vi "Zone-to-color_correspondence_lookup_test_2.vi"() -> ()   [LabVIEW 2018]
uses:
  <userlib>/_OpenG.lib/array/array.llb/Sort 1D Array (U32)__ogtk.vi
  <userlib>/_OpenG.lib/array/array.llb/Index 1D Array Elements (U32)__ogtk.vi
  <vilib>/Analysis/polynomials.llb/Unique Numbers and Multiplicity (DBL).vi
  <userlib>/_OpenG.lib/array/array.llb/Index 1D Array Elements (DBL)__ogtk.vi
  <vilib>/Analysis/NI_AALPro.lvlib
panel:
  out "Seconds per MPix":dbl
  out "Amount of colors":cluster{"Amount":u32, "Color":u32}[](array[cluster])
  out "Array size":i32
  out "Image Display":T1(plugin-control)
  in  "Labyrinth path":path=path "D:/Users_Data/Dmitriy_T/Documents/Tracker/TestVI's/Labyrinth_check.png"
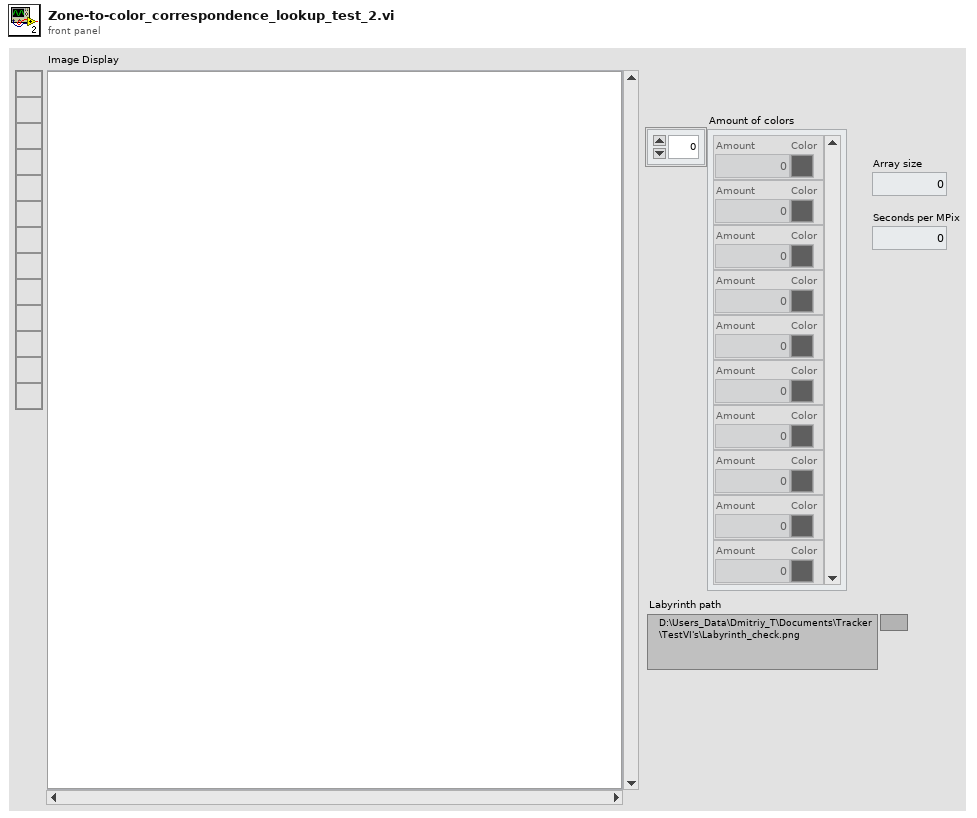
[diagram p1: front panel]
types:
  T1 = typedef "IMAQ Image.ctl" = refnum<image>
  T2 = typedef "Image Type" = u32
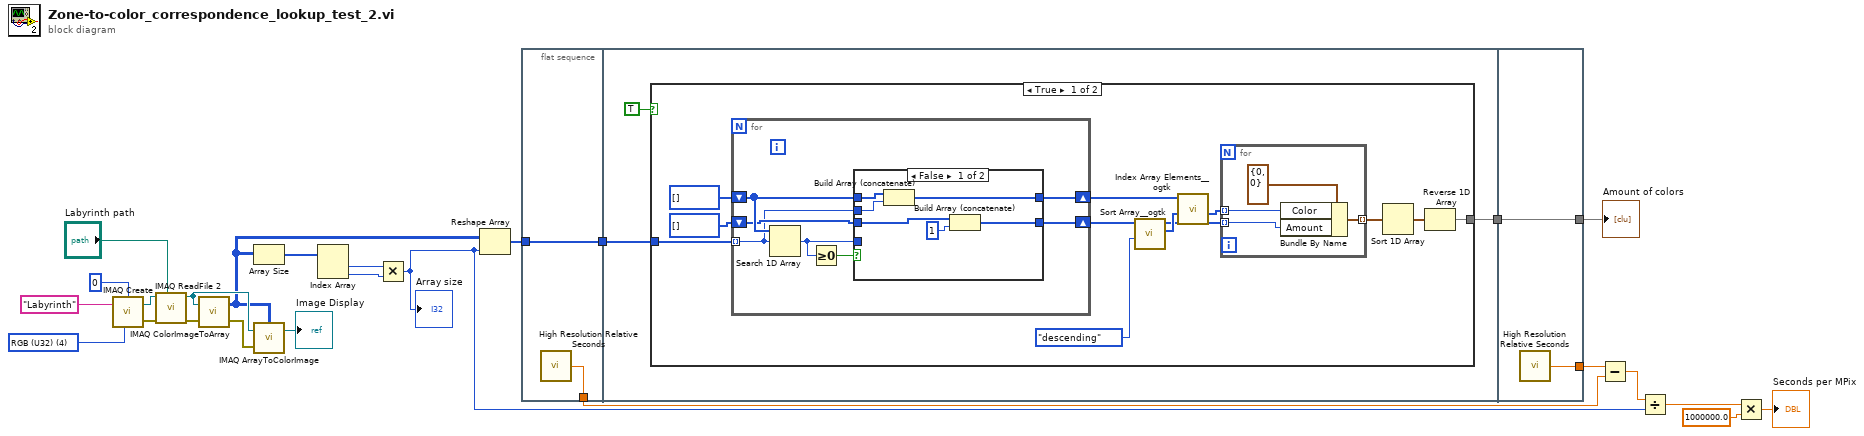
[diagram p0: block diagram]
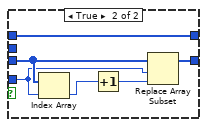
[diagram p2: hidden frame]
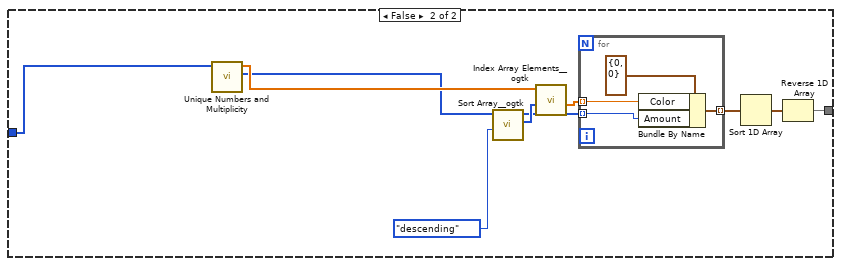
[diagram p3: hidden frame]
diagram:
  w16 = T2 4 items=["Grayscale (U8)", "Grayscale (I16)", "Grayscale (SGL)", "Complex (CSG)", "RGB (U32)", "HSL (U32)", "RGB (U64)", "Grayscale (U16)"] ("Image Type")
  n1 = call "IMAQ Create"("Border Size"=0, "Image Name"="Labyrinth", "Image Type"=w16) -> ("New Image"=w24:T1, "error out"=w22:errorcluster)  [unwired: 2 in]
  n2 = call "IMAQ ReadFile 2"("File Path"="Labyrinth path", "error in (no error)"=w22, "Image"=w24) -> ("error out"=w21:errorcluster, "Image Out"=w19:T1)  [unwired: 4 in, 3 out]
  n3 = call "IMAQ ColorImageToArray"("Image"=w19, "error in (no error)"=w21) -> ("Image Pixels (U32)"=w13:u32[][], "error out"=w18:errorcluster)  [unwired: 2 in, 1 out]
  n4 = Array Size(array=w13) -> (size(s)=w11:i32[])
  n5 = call "IMAQ ArrayToColorImage"("Image Pixels (U32)"=w13, "Image"=w19, "error in (no error)"=w18) -> ("Image Out"=→"Image Display":T1)  [unwired: 2 in, 1 out]
  n6 = Index Array(array=w11) -> (element #1=w15:i32, element #2=w14:i32)  [unwired: 2 in]
  n7 = Multiply(x=w15, y=w14) -> (x*y=w4:i32)
  "Array size" <- w4
  n8 = Reshape Array(w13, w4) -> (w10:u32[])
  n9 = flat-sequence {
    tunnel: w10 -> [w27]
    tunnel: [w27] -> w9
    tunnel: [w26] -> w6
    tunnel: w9 -> [w29]
    tunnel: [w30] -> w8
    tunnel: [w81] -> w12
    tunnel: w8 -> [w81]
    tunnel: [w80] -> w7
    frame #0 {
      n10 = call <vilib>:"High Resolution Relative Seconds.vi"() -> ("relative seconds"=w26:dbl)
    }
    frame #1 {
      n11 = case shown="True" TRUE {
        tunnel: [w40 w73] -> w30
        tunnel: w29 -> [w39 w68]
        frame True {
          n12 = for {
            tunnel: w39 -> [w43] mode=indexing
            shift-right: [w47] -> w34
            shift-left: u32[] [] -> [w48]
            shift-right: [w44] -> w35
            shift-left: u32[] [] -> [w46]
            n13 = Search 1D Array(1D array=w48, element=w43) -> (index of element=w45:i32)  [unwired: 1 in]
            n14 = Greater Or Equal To 0?(x=w45) -> (x >= 0?=w49:bool)
            n15 = case shown="False" w49 {
              tunnel: w48 -> [w55 w61]
              tunnel: [w54 w61] -> w47
              tunnel: w46 -> [w52 w60]
              tunnel: w45 -> [_ w59]
              tunnel: [w51 w56] -> w44
              tunnel: w43 -> [w53 _]
              frame False {
                n16 = Build Array (concatenate)(w55, w53) -> (w54:u32[])
                n17 = Build Array (concatenate)(w52, u32 1) -> (w51:u32[])
              }
              frame True {
                n18 = Index Array(array=w60, index=w59) -> (element=w58:u32)
                n19 = Increment(x=w58) -> (x+1=w57:u32)
                n20 = Replace Array Subset(array=w60, new element=w57, index=w59) -> (w56:u32[])
              }
            }
          }
          n21 = call-poly <userlib>:"Sort Array__ogtk.vi"("Order"=enum16{"ascending", "descending"}."descending", "Array in"=w35) -> ("Sorted Pointers"=w33:i32[], "Sorted Array out"=w31:u32[])  [unwired: 8 in]
          n22 = call-poly <userlib>:"Index Array Elements__ogtk.vi"("indices"=w33, "array"=w34) -> ("elements"=w32:u32[])  [unwired: 9 in]
          n23 = for {
            tunnel: w31 -> [w63] mode=indexing
            tunnel: w32 -> [w64] mode=indexing
            tunnel: [w62] -> w42 mode=indexing
            n24 = Bundle By Name(cluster=cluster{"Amount":u32, "Color":u32} {"Amount"=0, "Color"=0} ("Color amount"), "Color"=w64, "Amount"=w63) -> (w62:cluster{"Amount":u32, "Color":u32})
          }
          n25 = Sort 1D Array(array=w42) -> (sorted array=w41:cluster{"Amount":u32, "Color":u32}[])
          n26 = Reverse 1D Array(array=w41) -> (reversed array=w40:cluster{"Amount":u32, "Color":u32}[])
        }
        frame False {
          n27 = call-poly <vilib>:"Unique Numbers and Multiplicity.vi"("Numbers"=w68) -> ("Multiplicity"=w66:u32[], "Unique Numbers"=w67:dbl[])  [unwired: 8 in, 1 out]
          n28 = call-poly <userlib>:"Sort Array__ogtk.vi"("Order"=enum16{"ascending", "descending"}."descending", "Array in"=w66) -> ("Sorted Pointers"=w71:i32[], "Sorted Array out"=w69:u32[])  [unwired: 8 in]
          n29 = call-poly <userlib>:"Index Array Elements__ogtk.vi"("indices"=w71, "array"=w67) -> ("elements"=w70:dbl[])  [unwired: 9 in]
          n30 = for {
            tunnel: w69 -> [w77] mode=indexing
            tunnel: w70 -> [w78] mode=indexing
            tunnel: [w76] -> w75 mode=indexing
            n31 = Bundle By Name(cluster=cluster{"Amount":u32, "Color":u32} {"Amount"=0, "Color"=0} ("Color amount"), "Color"=w78, "Amount"=w77) -> (w76:cluster{"Amount":u32, "Color":u32})
          }
          n32 = Sort 1D Array(array=w75) -> (sorted array=w74:cluster{"Amount":u32, "Color":u32}[])
          n33 = Reverse 1D Array(array=w74) -> (reversed array=w73:cluster{"Amount":u32, "Color":u32}[])
        }
      }
    }
    frame #2 {
      n34 = call <vilib>:"High Resolution Relative Seconds.vi"() -> ("relative seconds"=w80:dbl)
    }
  }
  n35 = Subtract(x=w7, y=w6) -> (x-y=w5:dbl)
  n36 = Divide(x=w5, y=w4) -> (x/y=w3:dbl)
  n37 = Multiply(x=w3, y=1000000.0) -> (x*y=→"Seconds per MPix":dbl)
  "Amount of colors" <- w12
